vi "Fetch Measurement (Monitor Spectrum).vi"(8 "error in (no error)":errorcluster, 10 "Select Trace (1: Trace 1)":u16(ring)=1 items=["Trace 1"=1, "Trace 2"=2, "Trace 3"=3], 11 "VISA resource name":refnum<visa-resource-name>) -> (0 "error out":errorcluster, 1 "Monitor Spectrum":cluster{dbl, dbl, dbl[]}(graph), 2 "Measured Values":dbl[](array[numeric]) format="%#.6g", 3 "VISA resource name out":refnum<visa-resource-name>)   [LabVIEW 2014, in "Agilent ESA PSA Series.lvlib"]
doc: "Returns the results of the last measurement (Monitor Spectrum) and does not initiate data acquisition.\n\n<B>Note:</B>\n\nThis VI is only valid for the Monitor Spectrum functionality of the Phase Noise and Noise Figure personalities."
uses:
  Agilent ESA PSA Series.lvlib
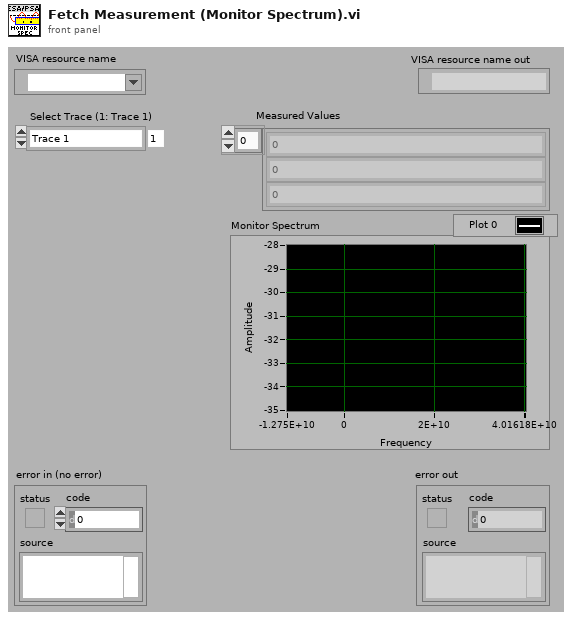
[diagram p1: front panel]
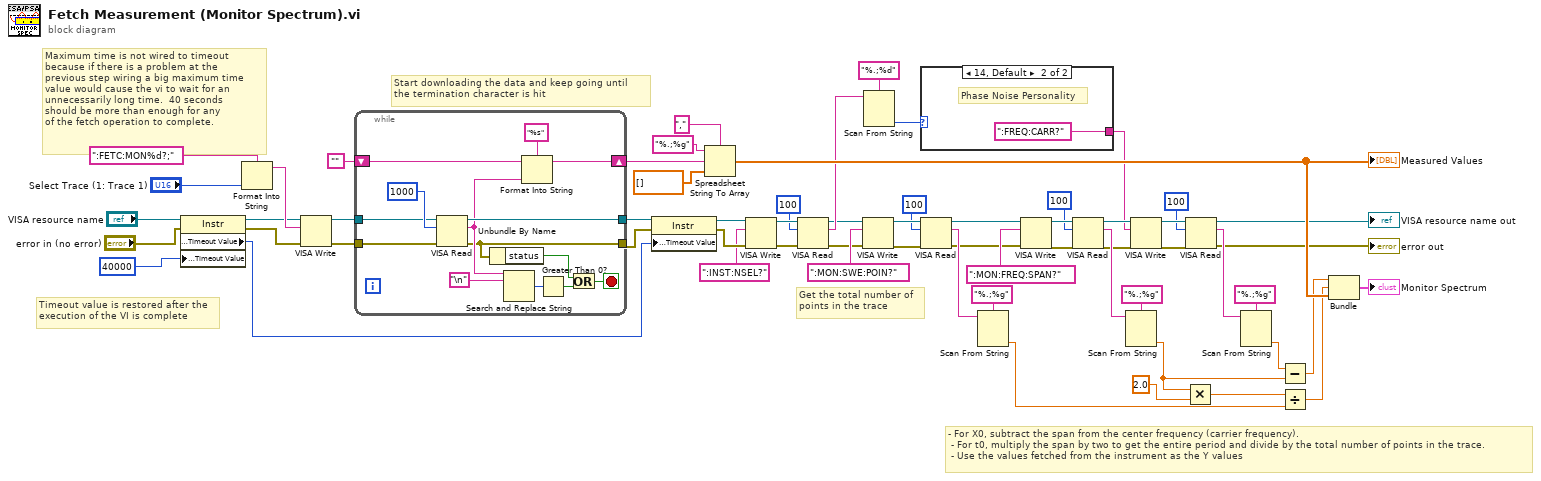
[diagram p0: block diagram]
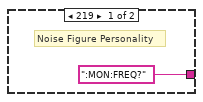
[diagram p2: hidden frame]
diagram:
  # "- For X0, subtract the span from the center frequency (carrier frequency). \n - For t0, multiply the span by two to get the entire period and divide by the total number of points in the trace.\n - Use the values fetched from the instrument as the Y values"
  # "Get the total number of\npoints in the trace"
  # "Maximum time is not wired to timeout\nbecause if there is a problem at the\nprevious step wiring a big maximum time\nvalue would cause the vi to wait for an\nunnecessarily long time.  40 seconds\nshould be more than enough for any\nof the fetch operation to complete."
  # "Timeout value is restored after the\nexecution of the VI is complete"
  # "Start downloading the data and keep going until\nthe termination character is hit"
  n1 = property on="Property Node" class="Instr"(reference="VISA resource name", error in="error in (no error)", "General Settings:Timeout Value"=u32 40000) -> (reference out=w57:refnum<visa-resource-name>, error out=w58:errorcluster, "General Settings:Timeout Value"=w54:u32)
  n2 = Format Into String(format string=":FETC:MON%d?;" ("string (\"\")"), "Select Trace (1: Trace 1)") -> (resulting string=w61:string)  [unwired: 2 in, 1 out]
  n3 = VISA Write(VISA resource name=w57, write buffer=w61, error in (no error)=w58) -> (VISA resource name out=w49:refnum<visa-resource-name>, error out=w48:errorcluster)  [unwired: 1 out]
  n4 = while {
    tunnel: [w75] -> w56
    tunnel: [w63] -> w55
    tunnel: w49 -> [w74]
    tunnel: w48 -> [w73]
    shift-right: [w69] -> w46
    shift-left: "" -> [w68]
    stop <- w64 stop-if-true
    n5 = VISA Read(VISA resource name=w74, byte count=u32 1000, error in (no error)=w73) -> (VISA resource name out=w75:refnum<visa-resource-name>, read buffer=w70:string, error out=w63:errorcluster)  [unwired: 1 out]
    n6 = Unbundle By Name(w63) -> ("status"=w66:bool)
    n7 = Search and Replace String(input string=w70, search string="\n") -> (number of replacements=w71:i32)  [unwired: 6 in, 3 out]
    n8 = Format Into String(format string="%s", initial string=w68, w70) -> (resulting string=w69:string)  [unwired: 1 in, 1 out]
    n9 = Greater Than 0?(x=w71) -> (x > 0?=w65:bool)
    n10 = Or(x=w66, y=w65) -> (x .or. y?=w64:bool)
  }
  n11 = property on="Property Node" class="Instr"(reference=w56, error in=w55, "General Settings:Timeout Value"=w54) -> (reference out=w12:refnum<visa-resource-name>, error out=w11:errorcluster)
  n12 = Spreadsheet String To Array(delimiter (Tab)=",", format string="%.;%g", spreadsheet string=w46, array type (2D Dbl)=dbl[] []) -> (array=w22:dbl[])
  "Measured Values" <- w22
  n13 = VISA Write(VISA resource name=w12, write buffer=":INST:NSEL?", error in (no error)=w11) -> (VISA resource name out=w9:refnum<visa-resource-name>, error out=w8:errorcluster)  [unwired: 1 out]
  n14 = VISA Read(VISA resource name=w9, byte count=u32 100, error in (no error)=w8) -> (VISA resource name out=w2:refnum<visa-resource-name>, read buffer=w5:string, error out=w1:errorcluster)  [unwired: 1 out]
  n15 = VISA Write(VISA resource name=w2, write buffer=":MON:SWE:POIN?", error in (no error)=w1) -> (VISA resource name out=w31:refnum<visa-resource-name>, error out=w30:errorcluster)  [unwired: 1 out]
  n16 = Scan From String(format string="%.;%d", input string=w5) -> (output 1=w6:i32)  [unwired: 3 in, 3 out]
  n17 = case shown="14, Default" w6 {
    tunnel: [":MON:FREQ?" ":FREQ:CARR?"] -> w3
    frame 219 {
      # "Noise Figure Personality"
    }
    frame 14, Default {
      # "Phase Noise Personality"
    }
  }
  n18 = VISA Read(VISA resource name=w31, byte count=u32 100, error in (no error)=w30) -> (VISA resource name out=w15:refnum<visa-resource-name>, read buffer=w27:string, error out=w16:errorcluster)  [unwired: 1 out]
  n19 = Scan From String(format string="%.;%g", input string=w27) -> (output 1=w19:dbl)  [unwired: 3 in, 3 out]
  n20 = VISA Write(VISA resource name=w15, write buffer=":MON:FREQ:SPAN?", error in (no error)=w16) -> (VISA resource name out=w43:refnum<visa-resource-name>, error out=w42:errorcluster)  [unwired: 1 out]
  n21 = VISA Read(VISA resource name=w43, byte count=u32 100, error in (no error)=w42) -> (VISA resource name out=w39:refnum<visa-resource-name>, read buffer=w40:string, error out=w38:errorcluster)  [unwired: 1 out]
  n22 = Scan From String(format string="%.;%g", input string=w40) -> (output 1=w23:dbl)  [unwired: 3 in, 3 out]
  n23 = VISA Write(VISA resource name=w39, write buffer=w3, error in (no error)=w38) -> (VISA resource name out=w37:refnum<visa-resource-name>, error out=w36:errorcluster)  [unwired: 1 out]
  n24 = Multiply(x=w23, y=2.0) -> (x*y=w18:dbl)
  n25 = VISA Read(VISA resource name=w37, byte count=u32 100, error in (no error)=w36) -> (VISA resource name out=→"VISA resource name out":refnum<visa-resource-name>, read buffer=w34:string, error out=→"error out":errorcluster)  [unwired: 1 out]
  n26 = Scan From String(format string="%.;%g", input string=w34) -> (output 1=w24:dbl)  [unwired: 3 in, 3 out]
  n27 = Subtract(x=w24, y=w23) -> (x-y=w20:dbl)
  n28 = Divide(x=w18, y=w19) -> (x/y=w17:dbl)
  n29 = Bundle(w20, w17, w22) -> (→"Monitor Spectrum":cluster{dbl, dbl, dbl[]})  [unwired: 1 in]
